vi "Go To Position (um).vi"(8 "error in (no error)":errorcluster, 10 "Position (um)":dbl[unit] format="%#_7g", 11 "GPIB # (in): def. 6":string="6") -> (0 "error out":errorcluster, 1 "coarse axis(steps)":dbl format="%#_7g", 2 "coarse axis (um)":ext[unit] format="%#_7g", 3 "GPIB # (out)":string, 4 "combined position (um)":ext[unit] format="%#_7g", 5 "fine axis (steps)":dbl format="%#_7g", 7 "fine axis (um)":ext[unit] format="%#_7g")   [LabVIEW 2009]
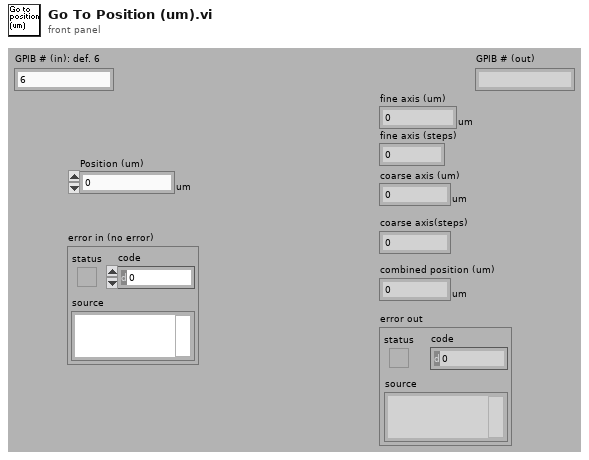
[diagram p1: front panel]
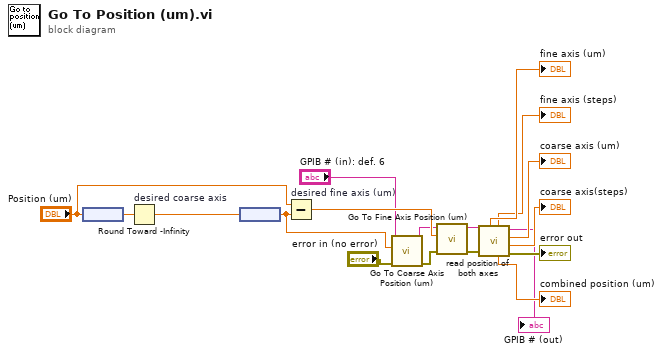
[diagram p0: block diagram]
diagram:
  n1 = node("Position (um)") -> (w16:dbl)
  n2 = Round Toward -Infinity "desired coarse axis"(1:w16) -> (0:w17:dbl)
  n3 = node(w17) -> (w18:dbl[unit])
  n4 = Subtract "desired fine axis (um)"(x="Position (um)", y=w18) -> (x-y=w9:dbl[unit])
  n5 = call "Go To Coarse Axis Position (um).vi"("error in (no error)"="error in (no error)", "Coarse Axis Position (um)"=w18, "GPIB # (in): def. 6"="GPIB # (in): def. 6") -> ("error out"=w8:errorcluster, "GPIB # (out)"=w3:string)  [unwired: 7 out]
  n6 = call "Go To Fine Axis Position (um).vi"("error in"=w8, "Fine Axis Position (um)"=w9, "GPIB # (in): def. 6"=w3) -> ("error out"=w7:errorcluster, "GPIB # (out)"=w4:string)  [unwired: 7 out]
  n7 = call "read position of both axes.vi"("GPIB # (in): def. 6"=w4, "error in (no error)"=w7) -> ("fine axis (um)"=→"fine axis (um)":ext[unit], "fine axis (steps)"=→"fine axis (steps)":dbl, "GPIB # (out)"=→"GPIB # (out)":string, "coarse axis (um)"=→"coarse axis (um)":ext[unit], "combined position (um)"=→"combined position (um)":ext[unit], "coarse axis(steps)"=→"coarse axis(steps)":dbl, "error out"=→"error out":errorcluster)  [unwired: 2 out]
